vi "ASIC_WRITE THX THX3 READ ADC.vi"(0 "ftHandle_in":u32, 1 "Sumador":u8, 2 "THX":u16, 3 "THX+3":u16, 5 "error in":errorcluster, 8 "Espera acceso USB 2":u32) -> (14 "ftHandle_out":u32, 16 "HLTHx":dbl, 17 "LLTHx":dbl, 19 "error out":errorcluster)   [LabVIEW 2019]
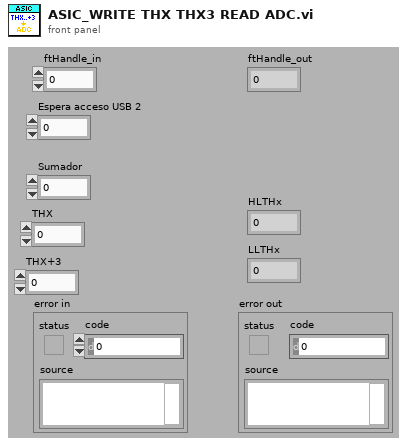
[diagram p1: front panel]
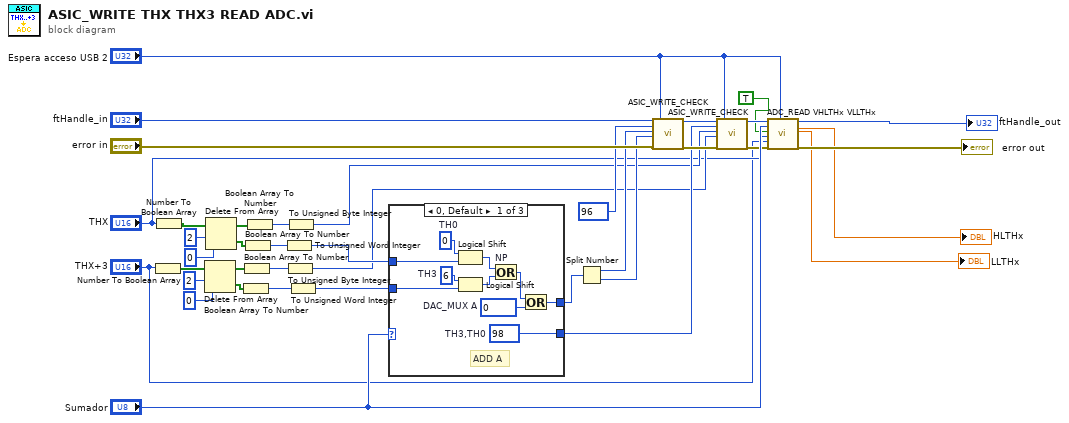
[diagram p0: block diagram]
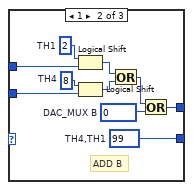
[diagram p2: hidden frame]
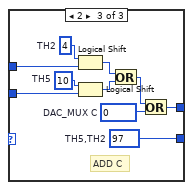
[diagram p3: hidden frame]
diagram:
  n1 = Number To Boolean Array(number="THX+3") -> (Boolean array=w16:bool[])
  n2 = Number To Boolean Array(number="THX") -> (Boolean array=w21:bool[])
  n3 = Delete From Array(array=w16, length=2, index=0) -> (deleted portion=w25:bool[], array with subset deleted=w24:bool[])
  n4 = Delete From Array(array=w21, length=2, index=0) -> (deleted portion=w23:bool[], array with subset deleted=w22:bool[])
  n5 = Boolean Array To Number(Boolean array=w25) -> (number=w27:u32)
  n6 = Boolean Array To Number(Boolean array=w24) -> (number=w29:u32)
  n7 = Boolean Array To Number(Boolean array=w23) -> (number=w26:u32)
  n8 = Boolean Array To Number(Boolean array=w22) -> (number=w28:u32)
  n9 = To Unsigned Word Integer(number=w26) -> (unsigned 16bit integer=w37:u16)
  n10 = To Unsigned Byte Integer(number=w29) -> (unsigned 8bit integer=w4:u8)
  n11 = To Unsigned Byte Integer(number=w28) -> (unsigned 8bit integer=w5:u8)
  n12 = To Unsigned Word Integer(number=w27) -> (unsigned 16bit integer=w38:u16)
  n13 = case shown="0, Default" "Sumador" {
    tunnel: [w48 w58 w68] -> w6
    tunnel: w37 -> [w47 w57 w67]
    tunnel: w38 -> [w46 w56 w66]
    tunnel: [w40 w50 w60] -> w9
    frame 0, Default {
      w39 = u16 0  # DAC_MUX A
      w44 = i8 6  # TH3
      w45 = i8 0  # TH0
      w48 = u8 98  # TH3,TH0
      # "ADD A"
      n14 = Logical Shift(y=w45, x=w47) -> (x << y=w42:u16)
      n15 = Logical Shift(y=w44, x=w46) -> (x << y=w43:u16)
      n16 = Or "NP"(x=w42, y=w43) -> (x .or. y?=w41:u16)
      n17 = Or(x=w41, y=w39) -> (x .or. y?=w40:u16)
    }
    frame 1 {
      w49 = u16 0  # DAC_MUX B
      w54 = i8 8  # TH4
      w55 = i8 2  # TH1
      w58 = u8 99  # TH4,TH1
      # "ADD B"
      n18 = Logical Shift(y=w55, x=w57) -> (x << y=w52:u16)
      n19 = Logical Shift(y=w54, x=w56) -> (x << y=w53:u16)
      n20 = Or(x=w52, y=w53) -> (x .or. y?=w51:u16)
      n21 = Or(x=w51, y=w49) -> (x .or. y?=w50:u16)
    }
    frame 2 {
      w59 = u16 0  # DAC_MUX C
      w64 = i8 10  # TH5
      w65 = i8 4  # TH2
      w68 = u8 97  # TH5,TH2
      # "ADD C"
      n22 = Logical Shift(y=w65, x=w67) -> (x << y=w62:u16)
      n23 = Logical Shift(y=w64, x=w66) -> (x << y=w63:u16)
      n24 = Or(x=w62, y=w63) -> (x .or. y?=w61:u16)
      n25 = Or(x=w61, y=w59) -> (x .or. y?=w60:u16)
    }
  }
  n26 = Split Number(x=w9) -> (hi(x)=w11:u8, lo(x)=w12:u8)
  n27 = call "ASIC_WRITE_CHECK.vi"("ftHandle_in"="ftHandle_in", "Direccion Registro Asic"=u8 96, "Byte Alto"=w11, "Byte Bajo"=w12, "error in"="error in", "Espera acceso USB 2"="Espera acceso USB 2") -> ("ftHandle_out"=w7:u32, "error out"=w8:errorcluster)  [unwired: 11 in, 1 out]
  n28 = call "ASIC_WRITE_CHECK.vi"("ftHandle_in"=w7, "Direccion Registro Asic"=w6, "Byte Alto"=w5, "Byte Bajo"=w4, "error in"=w8, "Espera acceso USB 2"="Espera acceso USB 2") -> ("ftHandle_out"=w13:u32, "error out"=w14:errorcluster)  [unwired: 11 in, 1 out]
  n29 = call "ADC_READ VHLTHx VLLTHx.vi"("ftHandle_out 2"=w13, "Sumador"="Sumador", "referenciar"=TRUE, "ref DAC\nTH0,TH1,TH2"="THX", "ref DAC\nTH3,TH4,TH5"="THX+3", "error out 2"=w14, "Espera acceso FT"="Espera acceso USB 2") -> ("ftHandle_out"=→"ftHandle_out":u32, "HLTHx"=→"HLTHx":dbl, "LLTHx"=→"LLTHx":dbl, "error out"=→"error out":errorcluster)  [unwired: 8 in, 1 out]
